vi "ZonalValues.vi"(8 "error in (no error)":errorcluster, 10 "HasoSlopes In":refnum<class "HasoSlopes.lvclass">, 11 "HASO4_3 in":refnum<class "HASO4_3.lvclass">) -> (0 "error out":errorcluster, 2 "HasoSlopesOut":refnum<class "HasoSlopes.lvclass">, 3 "HASO4_3 out":refnum<class "HASO4_3.lvclass">, 4 "Pamameter":T1, 6 "StatisticsData":T2)   [LabVIEW 2020, in "HASO4_3.lvclass"]
uses:
  HASO4_3.lvclass
  HasoSlopes.lvclass
  StatisticsData.ctl
  Pupil.lvclass
  Phase.lvclass
  HasoData.lvclass
  ComputePhaseSet.lvclass
  Point2Df.ctl
  WavefrontReconstructionMode.ctl
  HASO4_3.lvclass/HASO4_3.ctl
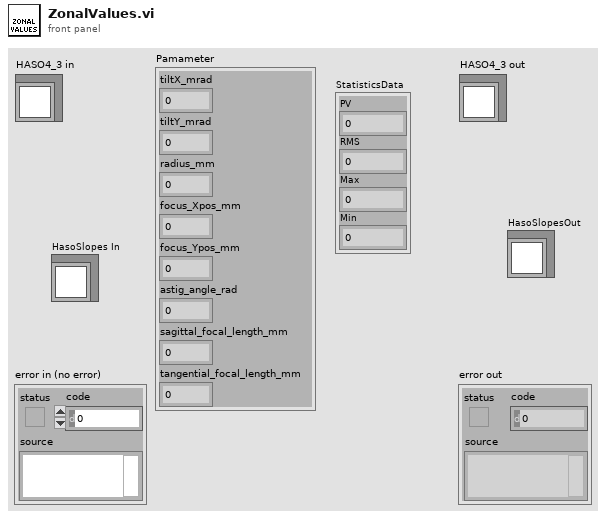
[diagram p1: front panel]
types:
  T1 = cluster{"tiltX_mrad":sgl, "tiltY_mrad":dbl, "radius_mm":sgl, "focus_Xpos_mm":sgl, "focus_Ypos_mm":sgl, "astig_angle_rad":sgl, "sagittal_focal_length_mm":sgl, "tangential_focal_length_mm":sgl}
  T2 = typedef "StatisticsData.ctl" = cluster{"PV":sgl, "RMS":dbl, "Max":sgl, "Min":sgl}
  T3 = typedef "WavefrontReconstructionMode.ctl" = enum16{"None", "Modal_Legendre", "Modal_Zernike", "Zonal", "Modal_Zonal_Zernike", "Modal_Zonal_Legendre"}
  T4 = typedef "Point2Df.ctl" = cluster{"X":sgl, "Y":sgl}
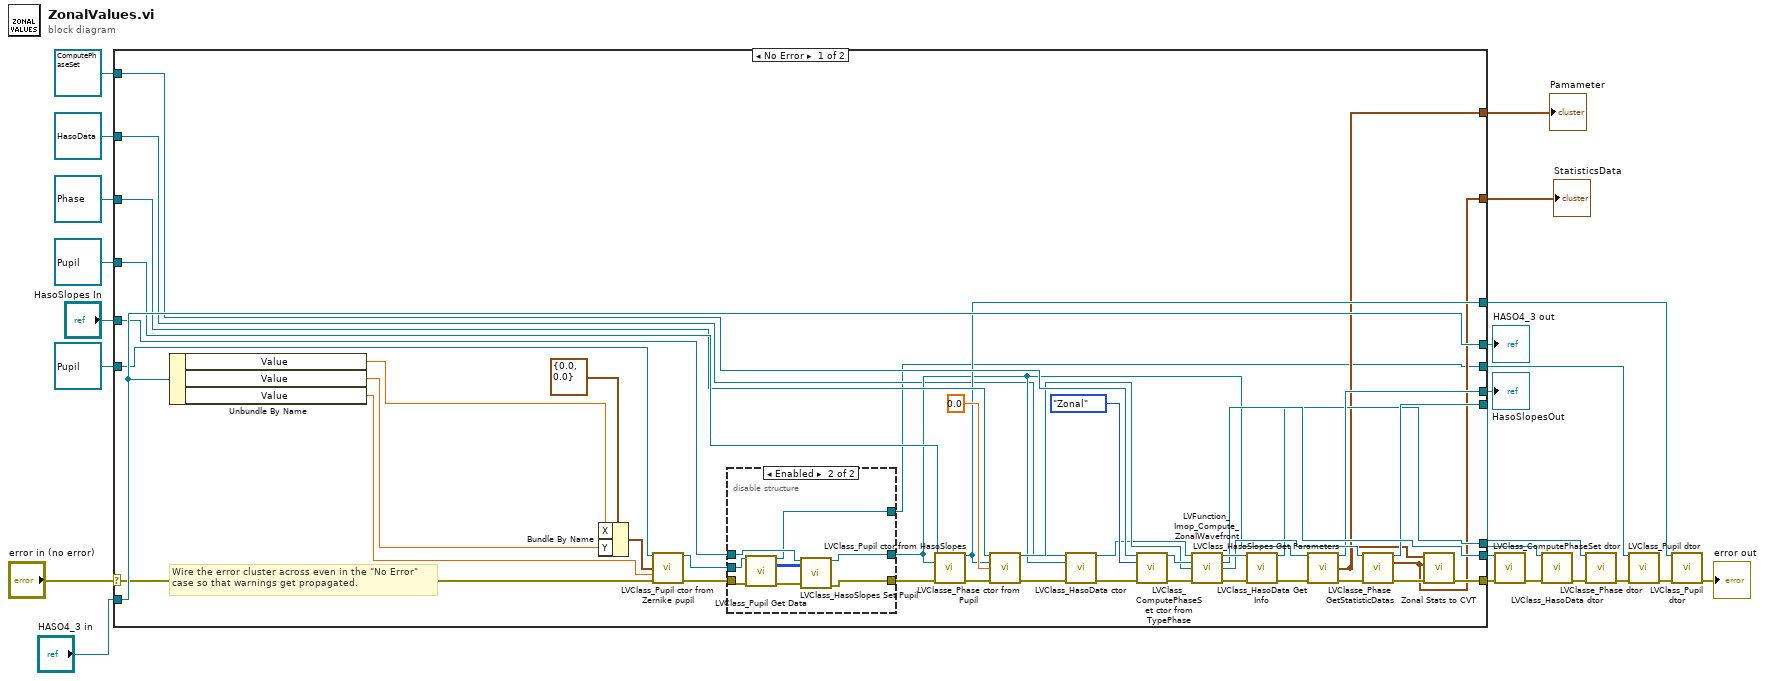
[diagram p0: block diagram]
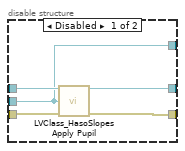
[diagram p2: hidden frame]
diagram:
  n1 = case shown="No Error" "error in (no error)" {
    selector: "error in (no error)" -> [w34 w85]
    tunnel: [w32 w85] -> w10
    tunnel: [w64 w84] -> w21
    tunnel: "HASO4_3 in" -> [w64 w84]
    tunnel: "HasoSlopes In" -> [w60 w82]
    tunnel: refnum<class "Pupil.lvclass"> refnum ("Pupil.lvclass") -> [w59 w83]
    tunnel: refnum<class "Pupil.lvclass"> refnum ("Pupil.lvclass") -> [w55 w78]
    tunnel: refnum<class "Phase.lvclass"> refnum ("Phase.lvclass") -> [w54 w80]
    tunnel: refnum<class "HasoData.lvclass"> refnum ("HasoData.lvclass") -> [w28 w79]
    tunnel: refnum<class "ComputePhaseSet.lvclass"> refnum ("ComputePhaseSet.lvclass") -> [w49 w81]
    tunnel: [w41 w81] -> w14
    tunnel: [w40 w82] -> w4
    tunnel: [w24 w83] -> w13
    tunnel: [w38 w78] -> w12
    tunnel: [w37 w80] -> w8
    tunnel: [w35 w79] -> w11
    tunnel: [w26 _] -> w2
    tunnel: [w25 _] -> w1
    frame No Error {
      # "Wire the error cluster across even in the \"No Error\"\ncase so that warnings get propagated."
      n2 = Unbundle By Name(w64) -> ("Value"=w62:dbl, "Value"=w61:dbl, "Value"=w57:dbl)
      n3 = Bundle By Name(cluster=T4 {"X"=0.0, "Y"=0.0} ("Pupil Dims.center"), "X"=w62, "Y"=w61) -> (w58:T4)
      n4 = call "LVClass_Pupil ctor from Zernike pupil.vi"("Pupil (const)"=w59, "center"=w58, "rayon"=w57, "error constant"=w34) -> ("Pupil (new)"=w39:refnum<class "Pupil.lvclass">, "error IO"=w56:errorcluster)  [unwired: 10 in]
      n5 = disable-structure shown="Enabled" {
        disable-tunnel: w60 -> [w69 w74]
        disable-tunnel: w56 -> [w68 w76]
        disable-tunnel: [w67 w72] -> w52
        disable-tunnel: w39 -> [w65 w77]
        disable-tunnel: [w66 w71] -> w29
        disable-tunnel: [w65 w70] -> w24
        frame Disabled {
          n6 = call "LVClass_HasoSlopes Apply Pupil.vi"("HasoSlopes in"=w69, "Pupil IN"=w65, "error in (no error)"=w68) -> ("HasoSlopes out"=w66:refnum<class "HasoSlopes.lvclass">, "error out"=w67:errorcluster)  [unwired: 11 in]
        }
        frame Enabled {
          n7 = call "LVClass_Pupil Get Data.vi"("Pupil in"=w77, "error in (no error)"=w76) -> ("Pupil out"=w70:refnum<class "Pupil.lvclass">, "Data"=w75:i32[][], "error out"=w73:errorcluster)  [unwired: 11 in]
          n8 = call "LVClass_HasoSlopes Set Pupil.vi"("HasoSlopes in"=w74, "Pupil"=w75, "error in (no error)"=w73) -> ("HasoSlopes out"=w71:refnum<class "HasoSlopes.lvclass">, "error out"=w72:errorcluster)  [unwired: 11 in]
        }
      }
      n9 = call "LVClass_Pupil ctor from HasoSlopes.vi"("Pupil (const)"=w55, "HasoSlopes"=w29, "error in (no error)"=w52) -> ("Pupil (new)"=w38:refnum<class "Pupil.lvclass">, "error out"=w51:errorcluster)  [unwired: 10 in, 1 out]
      n10 = call "LVClasse_Phase ctor from Pupil.vi"("Phase (const)"=w54, "Pupil"=w38, "coef"=sgl 0.0, "error in (no error)"=w51) -> ("Phase (new)"=w47:refnum<class "Phase.lvclass">, "error out"=w31:errorcluster)  [unwired: 9 in, 1 out]
      n11 = call "LVClass_HasoData ctor.vi"("HasoData (const)"=w28, "HasoSlopes"=w29, "error in (no error)"=w31) -> ("HasoData (new)"=w27:refnum<class "HasoData.lvclass">, "error out"=w30:errorcluster)  [unwired: 10 in, 1 out]
      n12 = call "LVClass_ComputePhaseSet ctor from TypePhase.vi"("ComputePhaseSet (const)"=w49, "TypePhase"=WavefrontReconstructionMode."Zonal", "error in (no error)"=w30) -> ("ComputePhaseSet (new)"=w48:refnum<class "ComputePhaseSet.lvclass">, "error out"=w46:errorcluster)  [unwired: 11 in]
      n13 = call "LVFunction_Imop_Compute_ZonalWavefront.vi"("HasoData.lvclass"=w27, "ComputePhaseSet.lvclass"=w48, "Phase"=w47, "error constant"=w46) -> ("HasoData.lvclass (dup)"=w44:refnum<class "HasoData.lvclass">, "ComputePhaseSet.lvclass 2"=w41:refnum<class "ComputePhaseSet.lvclass">, "Phase"=w42:refnum<class "Phase.lvclass">, "error out"=w45:errorcluster)  [unwired: 8 in]
      n14 = call "LVClass_HasoData Get Info.vi"("HasoData in"=w44, "error in (no error)"=w45) -> ("HasoData out"=w35:refnum<class "HasoData.lvclass">, "error out"=w43:errorcluster)  [unwired: 11 in, 1 out]
      n15 = call "LVClass_HasoSlopes Get Parameters.vi"("HasoSlopes in"=w29, "error in (no error)"=w43) -> ("HasoSlopes out"=w40:refnum<class "HasoSlopes.lvclass">, "Pamameter"=w26:T1, "error out"=w36:errorcluster)  [unwired: 11 in]
      n16 = call "LVClasse_Phase GetStatisticDatas.vi"("Phase in"=w42, "error in (no error)"=w36) -> ("Phase out"=w37:refnum<class "Phase.lvclass">, "StatisticsData"=w25:T2, "error out"=w33:errorcluster)  [unwired: 11 in]
      n17 = call "Zonal Stats to CVT.vi"("error in (no error)"=w33, "StatisticsData"=w25, "Pamameter"=w26) -> ("error out"=w32:errorcluster)  [unwired: 8 in]
    }
    frame Error {
    }
  }
  "HASO4_3 out" <- w21
  "HasoSlopesOut" <- w4
  "Pamameter" <- w2
  "StatisticsData" <- w1
  n18 = call "LVClass_ComputePhaseSet dtor.vi"("ComputePhaseSet in"=w14, "error in (no error)"=w10) -> ("error out"=w9:errorcluster)  [unwired: 12 in, 1 out]
  n19 = call "LVClass_HasoData dtor.vi"("HasoData in"=w11, "error in (no error)"=w9) -> ("error out"=w3:errorcluster)  [unwired: 12 in, 1 out]
  n20 = call "LVClasse_Phase dtor.vi"("Phase in"=w8, "error in (no error)"=w3) -> ("error out"=w7:errorcluster)  [unwired: 12 in, 1 out]
  n21 = call "LVClass_Pupil dtor.vi"("Pupil in"=w13, "error in (no error)"=w7) -> ("error out"=w6:errorcluster)  [unwired: 12 in, 1 out]
  n22 = call "LVClass_Pupil dtor.vi"("Pupil in"=w12, "error in (no error)"=w6) -> ("error out"=→"error out":errorcluster)  [unwired: 12 in, 1 out]
